vi "Parse-attribute.vi"(8 "error in (no error)":errorcluster, 10 "String in":string, 11 "Speed in":refnum<class "Speed.lvclass">) -> (0 "error out":errorcluster, 1 "Valid attribute?":bool, 2 "Remaining string":string, 3 "Speed out":refnum<class "Speed.lvclass">)   [LabVIEW 2013, in "HardwareCharacterization.lvlib" / "Speed.lvclass"]
uses:
  Speed.lvclass
  Speed.lvclass/Speed.ctl
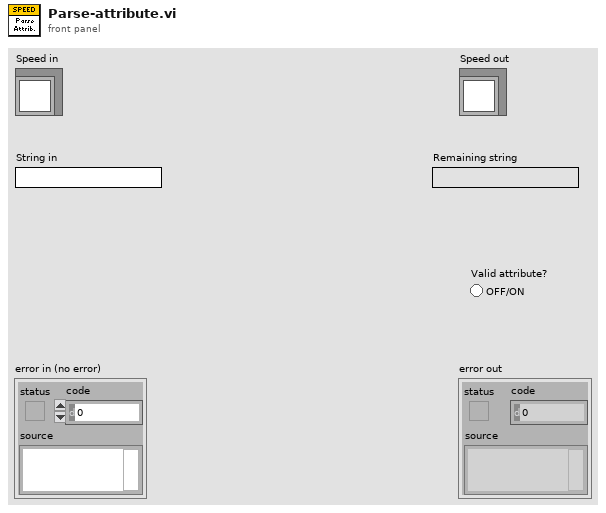
[diagram p1: front panel]
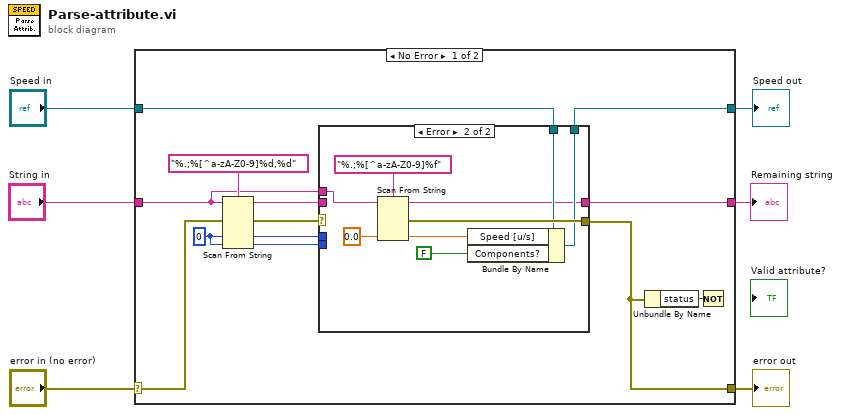
[diagram p0: block diagram]
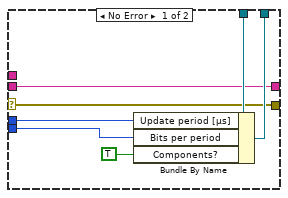
[diagram p2: hidden frame]
diagram:
  n1 = case shown="No Error" "error in (no error)" {
    selector: "error in (no error)" -> [w13 w38]
    tunnel: [w8 w38] -> w5
    tunnel: [w14 w37] -> w3
    tunnel: "Speed in" -> [w15 w37]
    tunnel: "String in" -> [w10 w36]
    tunnel: [w7 w36] -> w1
    frame No Error {
      w12 = u16 0 ("default value 2")
      n2 = Scan From String(format string="%.;%[^a-zA-Z0-9]%d,%d", input string=w10, error in=w13, default 2=w12, default 3=w12) -> (remaining string=w9:string, error out=w11:errorcluster, output 2=w17:u16, output 3=w16:u16)  [unwired: 3 in, 1 out]
      n3 = case shown="Error" w11 {
        selector: w11 -> [w22 _]
        tunnel: w17 -> [w26 _]
        tunnel: w16 -> [w25 _]
        tunnel: w15 -> [w24 w29]
        tunnel: [w23 w28] -> w14
        tunnel: [w22 w32] -> w8
        tunnel: w10 -> [_ w33]
        tunnel: w9 -> [w20 _]
        tunnel: [w20 w27] -> w7
        frame No Error {
          n4 = Bundle By Name(cluster=w24, "Update period [µs]"=w26, "Bits per period"=w25, "Components?"=TRUE) -> (w23:refnum<class "Speed.lvclass">)
        }
        frame Error {
          n5 = Scan From String(format string="%.;%[^a-zA-Z0-9]%f", input string=w33, default 2=0.0 ("default value 2")) -> (remaining string=w27:string, error out=w32:errorcluster, output 2=w31:dbl)  [unwired: 4 in, 1 out]
          n6 = Bundle By Name(cluster=w29, "Speed [u/s]"=w31, "Components?"=FALSE) -> (w28:refnum<class "Speed.lvclass">)
        }
      }
      n7 = Unbundle By Name(w8) -> ("status"=w18:bool)
      n8 = Not(x=w18) -> ()  [unwired: 1 out]
    }
    frame Error {
    }
  }
  "error out" <- w5
  "Speed out" <- w3
  "Remaining string" <- w1
